vi "PicoScope5000aExampleRapidBlockBulk.vi"() -> ()   [LabVIEW 2009]
doc: "This example demonstrates how to use the PicoScope Labview library to collect data using rapid block mode, retrieving the data values in bulk.\nThis example requires LabVIEW 9.0 or later."
panel:
  out "Analog Channels":cluster{i32, sgl, "Data (Volts)":dbl[]}[](graph)
  in  "Channel A Settings":T1 {"Bandwidth Limit" items=["Full", "20MHz"]; "Range" items=["10 mV", "20 mV", "50 mV", "100 mV", "200 mV", "500 mV", "1 V", "2 V", "5 V", "10 V", "20 V"]; "Coupling" items=["AC", "DC"]}
  in  "Rapid Block Acquisition Settings":T2 {"Down Sample Ratio" min=1 step=1; "Down-Sample Mode" items=["None", "Aggregate", "Decimate", "Average"]}
  out "Device Info":T3
  out "Properties Panel":T4 {"Max Total Capture Time Available (sec)" format="%.3p"; "Sample Frequency" format="%.3p"; "Sample Rate" format="%.3p"; "Max Samples Available" format="%.3p"; "Total Capture Time (sec)" format="%.3p"}
  in  "Trigger Settings":T5 {"Trigger Direction" items=["Rising", "Falling"]}
  out "2-channel USB 3.0 device on non-USB 3.0 Port":bool
  out "4-channel USB Powered":bool
  in  "Serial Number":string
  in  "Use Serial Number":bool
  out "Number of Samples \nPer Capture":u32
  in  "Resolution":i32(ring) items=["8-bit", "12-bit", "14-bit", "15-bit (max. 2 ch.)", "16-bit (max. 1 ch.)"]
  out "Capture Complete":bool
  in  "Run":bool
  in  "Capture Index":i16 min=0
  in  "stop":bool
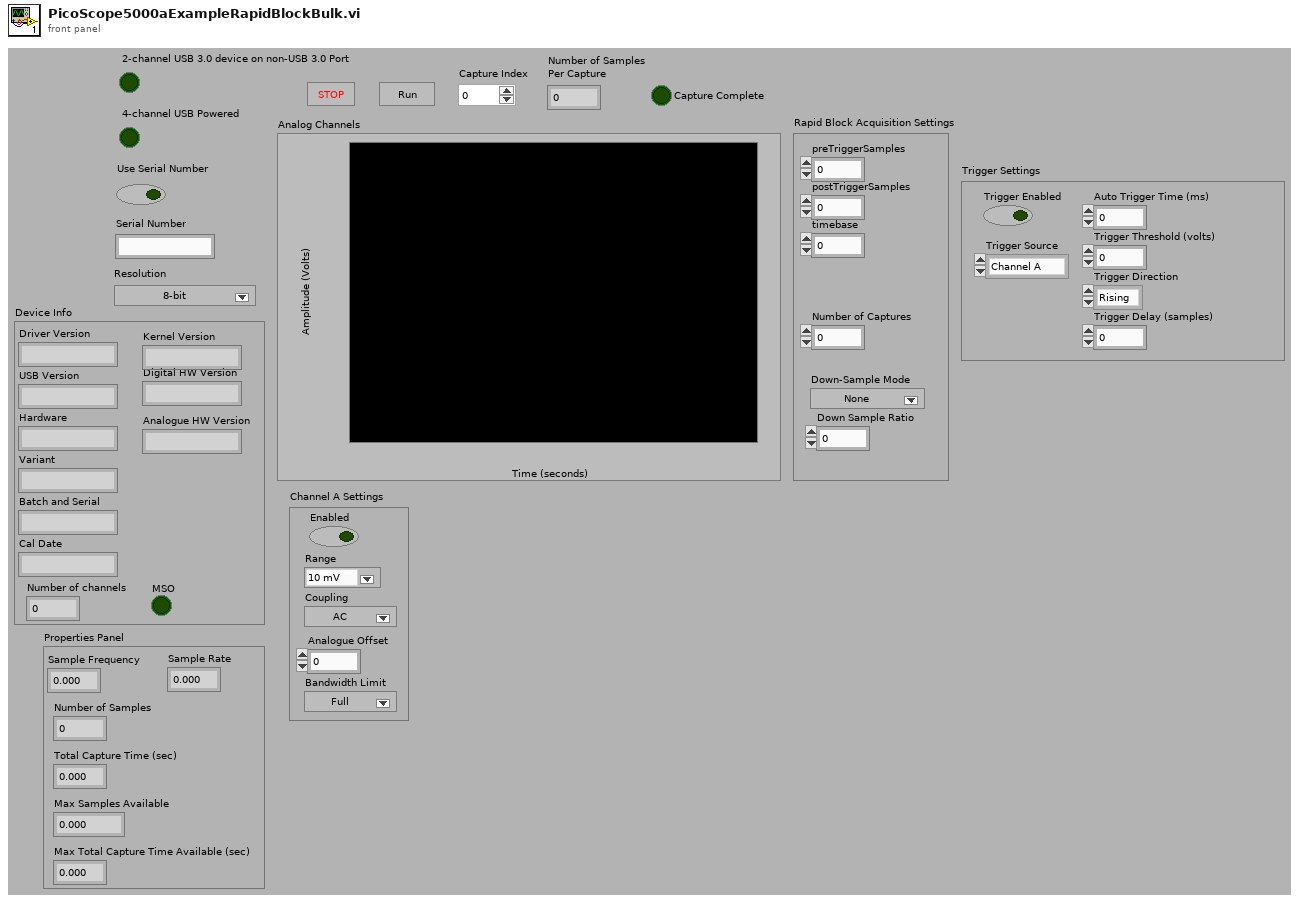
[diagram p1: front panel]
types:
  T1 = cluster{"Enabled":bool, "Coupling":i16, "Range":u16, "Analogue Offset":sgl, "Bandwidth Limit":u32}
  T2 = cluster{"preTriggerSamples":u32, "postTriggerSamples":u32, "timebase":u32, "Down-Sample Mode":i32, "Down Sample Ratio":u32, "Number of Captures":u32}
  T3 = cluster{"Driver Version":string, "USB Version":string, "Hardware":string, "Variant":string, "Batch and Serial":string, "Cal Date":string, "Kernel Version":string, "Digital HW Version":string, "Analogue HW Version":string, "MSO":bool, "Number of channels":i16}
  T4 = cluster{"Sample Frequency":sgl, "Sample Rate":sgl, "Max Samples Available":i32, "Number of Samples":u32, "Total Capture Time (sec) ":sgl, "Max Total Capture Time Available (sec)":sgl}
  T5 = cluster{"Trigger Enabled":bool, "Trigger Source":enum16{"Channel A", "Channel B", "Channel C", "Channel D", "Ext."}, "Trigger Threshold (volts)":dbl, "Trigger Direction":u16, "Trigger Delay (samples)":u32, "Auto Trigger Time (ms)":i16}
  T6 = cluster{"preTriggerSamples":u32, "postTriggerSamples":u32, "timebase":u32, "Down-Sample Mode":i32, "Down Sample Ratio":u32}
  T7 = cluster{i32, "Sample Rate":sgl, "Data (Volts)":dbl[]}
  T8 = cluster{i32, "Sample Rate":sgl, "Data (Volts)":dbl[]}[]
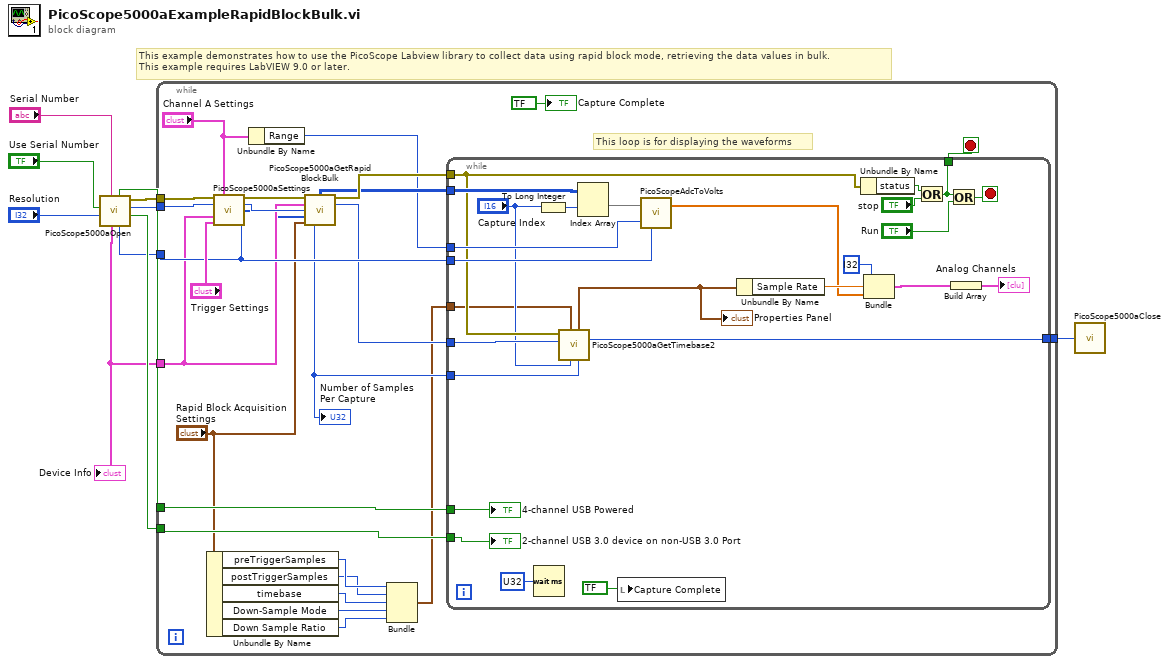
[diagram p0: block diagram]
diagram:
  # "This example demonstrates how to use the PicoScope Labview library to collect data using rapid block mode, retrieving the data values in bulk.\nThis example requires LabVIEW 9.0 or later."
  n1 = call "PicoScope5000aOpen.vi"("Serial Number"="Serial Number", "Resolution"="Resolution", "Use Serial Number"="Use Serial Number") -> ("USB Powered"=w7:bool, "handle"=w8:i16, "error out"=w9:errorcluster, "Max ADC value"=w2:i16, "USB 3.0 device on non-USB 3.0 Port"=w3:bool, "Device Info"=w1:T3)  [unwired: 3 in]
  "Device Info" <- w1
  n2 = while {
    tunnel: [w25] -> w10
    tunnel: w9 -> [w33]
    tunnel: w8 -> [w32]
    tunnel: w7 -> [w31]
    tunnel: w3 -> [w29]
    tunnel: w2 -> [w27]
    tunnel: w1 -> [w20]
    stop <- w36 stop-if-true
    # "This loop is for displaying the waveforms"
    n3 = Unbundle By Name("Rapid Block Acquisition Settings") -> ("preTriggerSamples"=w18:u32, "postTriggerSamples"=w17:u32, "timebase"=w15:u32, "Down-Sample Mode"=w14:i32, "Down Sample Ratio"=w13:u32)
    n4 = call "PicoScope5000aSettings.vi"("error in"=w33, "Channel A Settings"="Channel A Settings", "handle in"=w32, "Device Info"=w20, "Trigger Settings"="Trigger Settings", "Max ADC value"=w27) -> ("error out"=w24:errorcluster, "handle out"=w21:i16, "enabled array"=w12:i16[])  [unwired: 7 in]
    n5 = Unbundle By Name("Channel A Settings") -> ("Range"=w26:u16)
    n6 = call "PicoScope5000aGetRapidBlockBulk.vi"("error in"=w24, "Device Info"=w20, "handle in"=w21, "enabled array"=w12, "Rapid Block Acquisition Settings"="Rapid Block Acquisition Settings") -> ("Channel A Buffer"=w30:i16[][], "error out"=w34:errorcluster, "handle out"=w22:i16, "Num samples"=w23:u32)  [unwired: 2 in, 5 out]
    "Number of Samples \nPer Capture" <- w23
    n7 = Bundle("preTriggerSamples"=w18, "postTriggerSamples"=w17, "timebase"=w15, "Down-Sample Mode"=w14, "Down Sample Ratio"=w13) -> (w19:T6)  [unwired: 1 in]
    n8 = while {
      tunnel: [w61] -> w36
      tunnel: w30 -> [w55]
      tunnel: w34 -> [w47]
      tunnel: w31 -> [w39]
      tunnel: w29 -> [w40]
      tunnel: w27 -> [w54]
      tunnel: w26 -> [w53]
      tunnel: [w46] -> w25
      tunnel: w23 -> [w45]
      tunnel: w22 -> [w44]
      tunnel: w19 -> [w41]
      stop <- w60 stop-if-true
      n9 = Wait (ms)(milliseconds to wait=u32 ?) -> ()  [unwired: 1 out]
      n10 = To Long Integer(number="Capture Index") -> (32bit integer=w43:i32)
      n11 = call "PicoScope5000aGetTimebase2.vi"("Number of Samples"=w45, "Memory Segment"="Capture Index", "Acquisition Settings"=w41, "handle in"=w44, "error in (no error)"=w47) -> ("handle out"=w46:i16, "Properties Panel"=w48:T4)  [unwired: 4 in, 1 out]
      "Properties Panel" <- w48
      n12 = Index Array(array=w55, index (row)=w43) -> (element=w52:i16[])  [unwired: 1 in]
      n13 = local write "Capture Complete"(bool ? ("Capture Complete")) -> ()
      n14 = call "PicoScopeAdcToVolts.vi"("Max_adc"=w54, "Range Index"=w53, "Data"=w52) -> ("Data (Volts)"=w49:dbl[])
      n15 = Unbundle By Name(w48) -> ("Sample Rate"=w50:sgl)
      n16 = Unbundle By Name(w47) -> ("status"=w56:bool)
      n17 = Bundle(i32 ?, "Sample Rate"=w50, "Data (Volts)"=w49) -> (w37:T7)  [unwired: 1 in]
      n18 = Or(x=w56, y="stop") -> (x .or. y?=w61:bool)
      n19 = Or(x=w61, y="Run") -> (x .or. y?=w60:bool)
      n20 = Build Array(w37) -> (→"Analog Channels":T8)
      "4-channel USB Powered" <- w40
      "2-channel USB 3.0 device on non-USB 3.0 Port" <- w39
    }
    "Capture Complete" <- bool ? ("Capture Complete")
  }
  n21 = call "PicoScope5000aClose.vi"("handle"=w10) -> ()
